vi "PV HiLobe Pumps Control commands .vi"(8 "error in (no error)":errorcluster, 9 "HiLobe commands - Cluster":T1={"Parameter"=enum."Standby [002]", "Parameter\nread only<->describe"=FALSE, "off        on"=TRUE, "Control via interface"=1, "Configuration DO2 / DO1"=1} caption="Operating adjustment - Cluster" {"Control via interface" items=["remote"=1, "RS 485"=2, "PV.can"=4, "Key on front panel"=32, "Unlock the interface selection"=255]; "Configuration DO2 / DO1" items=["1 = no error"=1, "2 = error"=2, "5 = target speed is reached"=5, "6 = pump on"=6, "9 = \"0\""=9, "10 = \"1\""=10, "11 = remote priority active"=11]}, 10 "Adress of unit":u16=1 min=1 max=999 step=1, 11 "VISA session":refnum<visa-resource-name>) -> (0 "error out":errorcluster, 2 "response (data)":string, 3 "dup VISA session":refnum<visa-resource-name>)   [LabVIEW 2021, in "Pfeiffer Vacuum.lvlib"]
doc: "There are 8 parameters available, only one of which can be enabled at a time. \n\nStandby [002]\nFault acknowledgment [009]\nPump [010]\nCongiguration output DO2 [019]\nCongiguration output DO1 [024]\nSeed setting mode [026]\nControl via interface [060]\nInterface selection locked [061]\n\nNote: The controls right of this one will set the appropriate values for the selected parameter. Any settings for an parameter that is not selected will be ignored. If a value is out of range, it will be changed to either the upper or the lower limit of the range."
uses:
  <instrlib>/Pfeiffer Vacuum/Pfeiffer Vacuum.lvlib
  <instrlib>/Pfeiffer Vacuum/Public/HiLobe/PV HiLobe Control commands - Cluster.ctl
panel:
  # "Standby                                   \n Pump \n Speed setting mode \n  Interface selection locked"
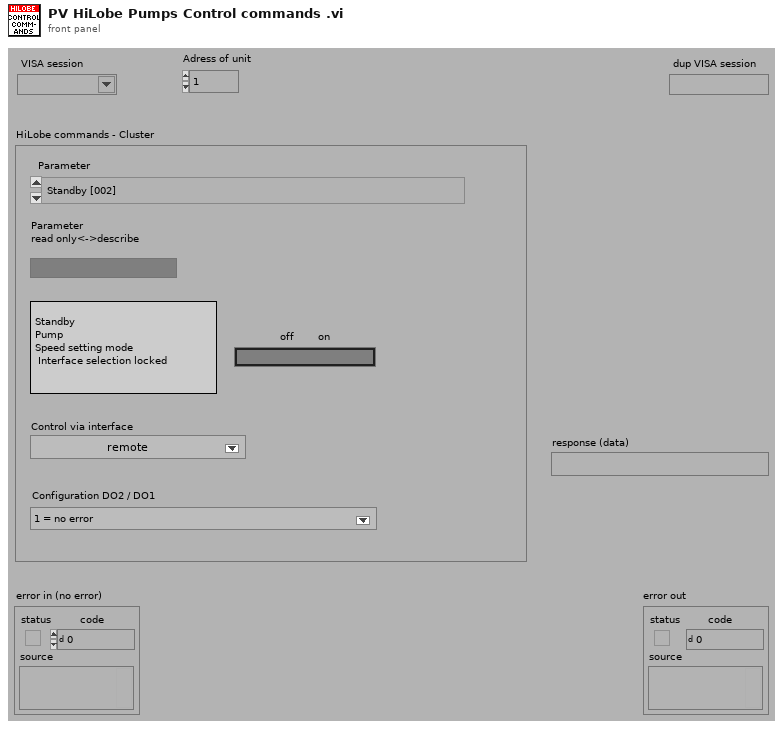
[diagram p1: front panel]
types:
  T1 = typedef "Pfeiffer Vacuum.lvlib/PV HiLobe Control commands - Cluster.ctl" = cluster{"Parameter":enum16{"Standby [002]", "Fault acknowledgment [009]", "Pump [010]", "Configuration output DO2 [019]", "Configuration output DO1 [024]", "Speed setting mode [026]", "Control via interface [060]", "Interface selection locked [061]"}, "Parameter\nread only<->describe":bool, "off        on":bool, "Control via interface":u16, "Configuration DO2 / DO1":u16}
  T2 = enum16{"Standby [002]", "Fault acknowledgment [009]", "Pump [010]", "Configuration output DO2 [019]", "Configuration output DO1 [024]", "Speed setting mode [026]", "Control via interface [060]", "Interface selection locked [061]"}
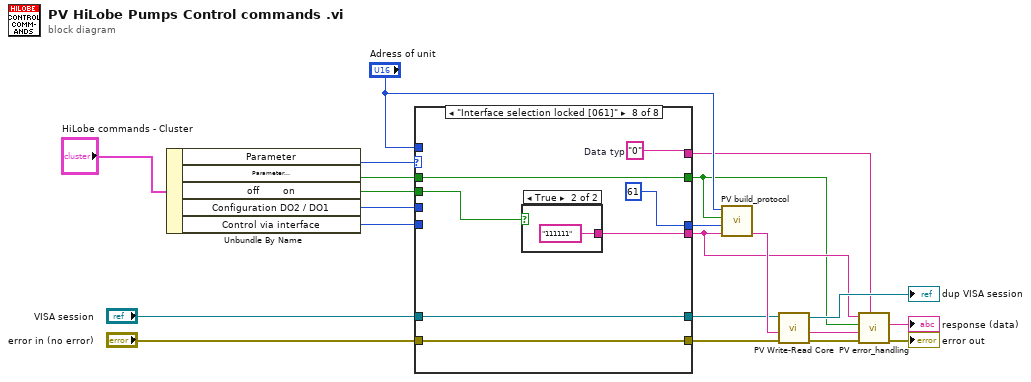
[diagram p0: block diagram]
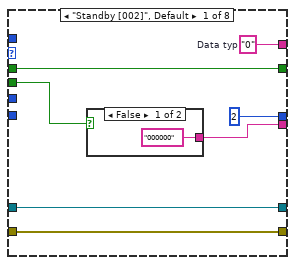
[diagram p2: hidden frame]
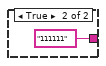
[diagram p3: hidden frame]
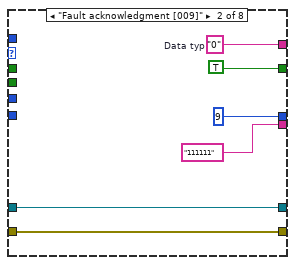
[diagram p4: hidden frame]
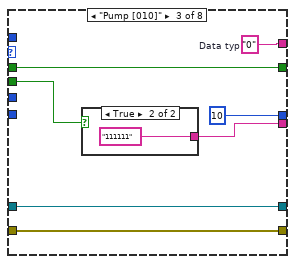
[diagram p5: hidden frame]
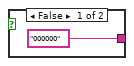
[diagram p6: hidden frame]
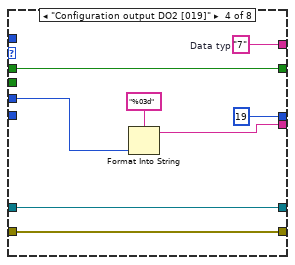
[diagram p7: hidden frame]
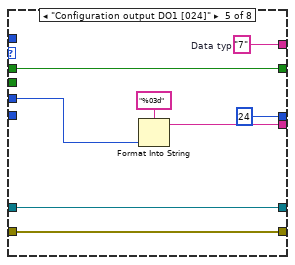
[diagram p8: hidden frame]
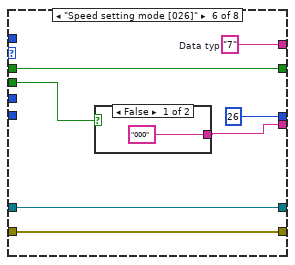
[diagram p9: hidden frame]
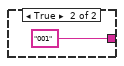
[diagram p10: hidden frame]
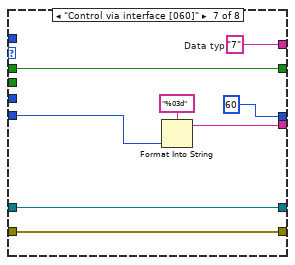
[diagram p11: hidden frame]
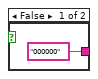
[diagram p12: hidden frame]
diagram:
  n1 = Unbundle By Name("HiLobe commands - Cluster") -> ("Parameter"=w20:T2, "Parameter\nread only<->describe"=w19:bool, "off        on"=w4:bool, "Configuration DO2 / DO1"=w3:u16, "Control via interface"=w2:u16)
  n2 = case shown="\"Interface selection locked [061]\"" w20 {
    tunnel: [u16 2 ("Parameter-number") u16 9 ("Parameter-number") u16 10 ("Parameter-number") u16 19 ("Parameter-number") u16 24 ("Parameter-number") u16 26 ("Parameter-number") u16 60 ("Parameter-number") u16 61 ("Parameter-number")] -> w21
    tunnel: [w27 "111111" ("Data") w42 w47 w55 w63 w72 w81] -> w9
    tunnel: [w26 TRUE w41 w53 w60 w64 w74 w80] -> w7
    tunnel: w19 -> [w26 _ w41 w53 w60 w64 w74 w80]
    tunnel: w4 -> [w25 _ w40 _ _ w62 _ w79]
    tunnel: [w24 w34 w39 w52 w59 w66 w75 w83] -> w8
    tunnel: "VISA session" -> [w23 w33 w38 w51 w58 w68 w78 w85]
    tunnel: [w23 w33 w38 w51 w58 w68 w78 w85] -> w14
    tunnel: "Adress of unit" -> [_ _ _ _ _ _ _ _]
    tunnel: "error in (no error)" -> [w22 w32 w37 w50 w57 w67 w77 w84]
    tunnel: [w22 w32 w37 w50 w57 w67 w77 w84] -> w13
    tunnel: w3 -> [_ _ _ w46 w54 _ _ _]
    tunnel: w2 -> [_ _ _ _ _ _ w71 _]
    frame "Standby [002]", Default {
      w24 = "0"  # Data typ
      n3 = case shown="False" w25 {
        tunnel: ["000000" ("Data") "111111" ("Data")] -> w27
        frame False {
        }
        frame True {
        }
      }
    }
    frame "Fault acknowledgment [009]" {
      w34 = "0"  # Data typ
    }
    frame "Pump [010]" {
      w39 = "0"  # Data typ
      n4 = case shown="True" w40 {
        tunnel: ["000000" ("Data") "111111" ("Data")] -> w42
        frame False {
        }
        frame True {
        }
      }
    }
    frame "Configuration output DO2 [019]" {
      w52 = "7"  # Data typ
      n5 = Format Into String(format string="%03d" ("Format-String"), w46) -> (resulting string=w47:string)  [unwired: 2 in, 1 out]
    }
    frame "Configuration output DO1 [024]" {
      w59 = "7"  # Data typ
      n6 = Format Into String(format string="%03d" ("Format-String"), w54) -> (resulting string=w55:string)  [unwired: 2 in, 1 out]
    }
    frame "Speed setting mode [026]" {
      w66 = "7"  # Data typ
      n7 = case shown="False" w62 {
        tunnel: ["000" ("Data") "001" ("Data")] -> w63
        frame False {
        }
        frame True {
        }
      }
    }
    frame "Control via interface [060]" {
      w75 = "7"  # Data typ
      n8 = Format Into String(format string="%03d" ("Format-String"), w71) -> (resulting string=w72:string)  [unwired: 2 in, 1 out]
    }
    frame "Interface selection locked [061]" {
      w83 = "0"  # Data typ
      n9 = case shown="True" w79 {
        tunnel: ["000000" ("Data") "111111" ("Data")] -> w81
        frame False {
        }
        frame True {
        }
      }
    }
  }
  n10 = call <instrlib>:"PV build_protocol.vi"("Data"=w9, "Parameter-number"=w21, "parameter\nread<->describe"=w7, "Adress"="Adress of unit") -> ("output"=w15:string)  [unwired: 3 in]
  n11 = call <instrlib>:"PV Write-Read Core.vi"("error in"=w13, "Write data in"=w15, "VISA session"=w14) -> ("error out"=w11:errorcluster, "response (data) out"=w12:string, "dup VISA session"=→"dup VISA session":refnum<visa-resource-name>)  [unwired: 2 in]
  n12 = call <instrlib>:"PV error_handling.vi"("Data Typ in"=w8, "error in"=w11, "response (data) in"=w12, "Parameter\nread only<->describe"=w7, "data in"=w9) -> ("error out"=→"error out":errorcluster, "Data out"=→"response (data)":string)  [unwired: 4 in, 1 out]
